vi "SIMULATION_SIM_ODOM_EXECUTE.vi"(8 "error in (no error)":errorcluster) -> (0 "error out":errorcluster)   [LabVIEW 2019]
uses:
  Swerve_Drive_System/SWERVE_DRIVE_GLOBALS.vi
  SIMULATION_SIM_Globals.vi
  <vilib>/Rock Robotics/WPI/ThirdParty/JAS_Junk/TrajLib/Trajectory_Library.lvlib
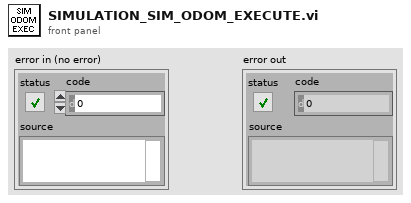
[diagram p1: front panel]
types:
  T1 = typedef "Trajectory_Library.lvlib/SWERVE_DRIVE_ODOMETRY.ctl" = cluster{"POSE":T2, "GyroOffset":T4, "PreviousAngle":T4, "PrevModulePositions":T5[], "NumModules":i32}
  T2 = typedef "Trajectory_Library.lvlib/POSE2D.ctl" = cluster{"TRANSLATION":T3, "ROTATION":T4}
  T3 = typedef "Trajectory_Library.lvlib/TRANSLATION2D.ctl" = cluster{"X":dbl, "Y":dbl}
  T4 = typedef "Trajectory_Library.lvlib/ROTATION2D.ctl" = cluster{"VALUE":dbl, "COS":dbl, "SIN":dbl}
  T5 = typedef "Trajectory_Library.lvlib/SWERVE_DRIVE_MODULE_POSITION.ctl" = cluster{"Distance":dbl, "Angle":T4, "P":bool}
  T6 = typedef "Trajectory_Library.lvlib/SWERVE_DRIVE_KINEMATICS.ctl" = cluster{"NumModules":i32, "InverseKinematics":T7, "ForwardKinematics":T7, "Modules":T3[], "PrevCoR":T3, "SavedModuleStates":T8[]}
  T7 = typedef "NI_Matrix.lvlib/RealMatrix.ctl" = dbl[][]
  T8 = typedef "Trajectory_Library.lvlib/SWERVE_DRIVE_MODULE_STATE.ctl" = cluster{"Speed":dbl, "Angle":T4}
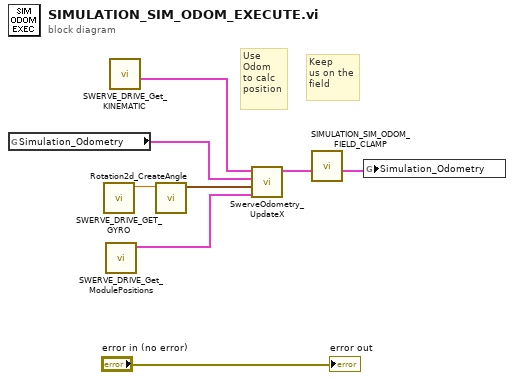
[diagram p0: block diagram]
diagram:
  # "Keep\nus on the\nfield"
  # "Use\nOdom\nto calc\nposition"
  n1 = global read "SIMULATION_SIM_Globals.vi" "Simulation_Odometry"() -> (w2:T1)
  n2 = call "SWERVE_DRIVE_GET_GYRO.vi"() -> ("Gyro Heading Radians"=w3:dbl)  [unwired: 11 in]
  n3 = call "SWERVE_DRIVE_Get_ModulePositions.vi"() -> ("Swerve Module Positions"=w5:T5[])  [unwired: 11 in]
  n4 = call "SWERVE_DRIVE_Get_KINEMATIC.vi"() -> ("out SWERVE_DRIVE_KINEMATICS"=w6:T6)  [unwired: 11 in]
  n5 = call <vilib>:"Rotation2d_CreateAngle.vi"("Angle"=w3) -> ("ROTATION"=w8:T4)  [unwired: 10 in]
  n6 = call <vilib>:"SwerveOdometry_UpdateX.vi"("module Positions"=w5, "gyroAngle"=w8, "in SWERVE_DRIVE_ODOMETRY"=w2, "SWERVE_DRIVE_KINEMATICS"=w6) -> ("out SWERVE_DRIVE_ODOMETRY"=w7:T1)  [unwired: 5 in, 2 out]
  n7 = call "SIMULATION_SIM_ODOM_FIELD_CLAMP.vi"("in SWERVE_DRIVE_ODOMETRY"=w7) -> ("out SWERVE_DRIVE_ODOMETRY"=w1:T1)  [unwired: 10 in]
  n8 = global write "SIMULATION_SIM_Globals.vi" "Simulation_Odometry"(w1) -> ()
  "error out" <- "error in (no error)"
